vi "Slack-Get Channel Users.vi"(0 "config in":T2, 11 "error in (no error)":errorcluster) -> (8 "users":T1[](array[typedef]), 15 "error out":errorcluster)   [LabVIEW 2015]
uses:
  Typedefs/Slack-Configuration.ctl
  Typedefs/Slack-User.ctl
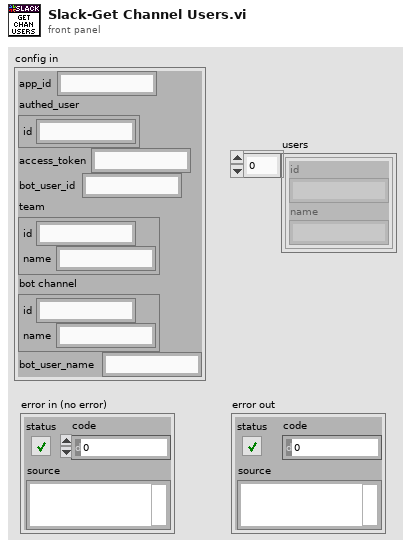
[diagram p1: front panel]
types:
  T1 = typedef "Slack-User.ctl" = cluster{"id":string, "name":string}
  T2 = typedef "Slack-Configuration.ctl" = cluster{"app_id":string, "authed_user":cluster{"id":string}, "access_token":string, "bot_user_id":string, "team":cluster{"id":string, "name":string}, "bot channel":cluster{"id":string, "name":string}, "bot_user_name":string}
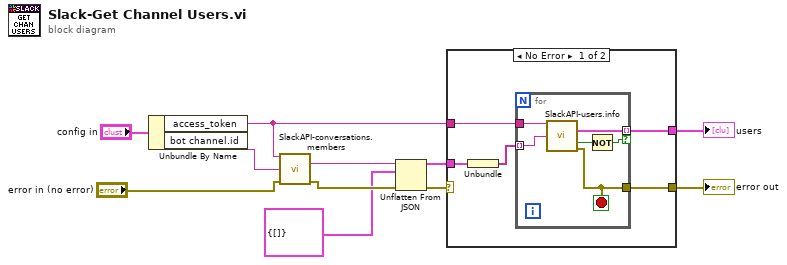
[diagram p0: block diagram]
diagram:
  n1 = Unbundle By Name("config in") -> ("access_token"=w2:string, "bot channel.id"=w11:string)
  n2 = call "SlackAPI-conversations.members.vi"("token"=w2, "id"=w11, "error in (no error)"="error in (no error)") -> ("body"=w10:string, "error out"=w9:errorcluster)  [unwired: 10 in, 1 out]
  n3 = Unflatten From JSON(JSON string=w10, type and defaults=cluster{"members":string[]} {"members"=[]}, error in (no error)=w9) -> (value=w8:cluster{"members":string[]}, error out=w7:errorcluster)  [unwired: 4 in]
  n4 = case shown="No Error" w7 {
    selector: w7 -> [_ w23]
    tunnel: w8 -> [w16 _]
    tunnel: [w13 w23] -> w5
    tunnel: w2 -> [w15 _]
    tunnel: [w12 _] -> w1
    frame No Error {
      n5 = Unbundle(w16) -> ("members"=w14:string[])
      n6 = for {
        tunnel: w15 -> [w22]
        tunnel: w14 -> [w21] mode=indexing
        tunnel: [w20] -> w13
        tunnel: [w19] -> w12 mode=indexing if=w18
        stop <- w20 stop-if-true
        n7 = call "SlackAPI-users.info.vi"("token"=w22, "user"=w21) -> ("user"=w19:T1, "is_bot"=w17:bool, "error out"=w20:errorcluster)  [unwired: 11 in]
        n8 = Not(x=w17) -> (.not. x?=w18:bool)
      }
    }
    frame Error {
    }
  }
  "error out" <- w5
  "users" <- w1
